vi "Get Joystick Values.vi"(8 "error in (no error)":errorcluster, 11 "Two Drivers in":refnum<class "Two Drivers.lvclass">) -> (0 "error out":errorcluster, 2 "Joystick Data":T1, 3 "Two Drivers out":refnum<class "Two Drivers.lvclass">)   [LabVIEW 2019, in "Joysticks.lvlib" / "Two Drivers.lvclass"]
doc: "Use this method to get the joystick values in a cluster you can use for your application.\n\nModify the Type Def that this VI resturns to fit the controls needed for the robot."
uses:
  Two Drivers.lvclass
  Joysticks.lvclass
  Controls/JoystickData.ctl
panel:
  in  "Sensitivity of Turret":dbl=45.0
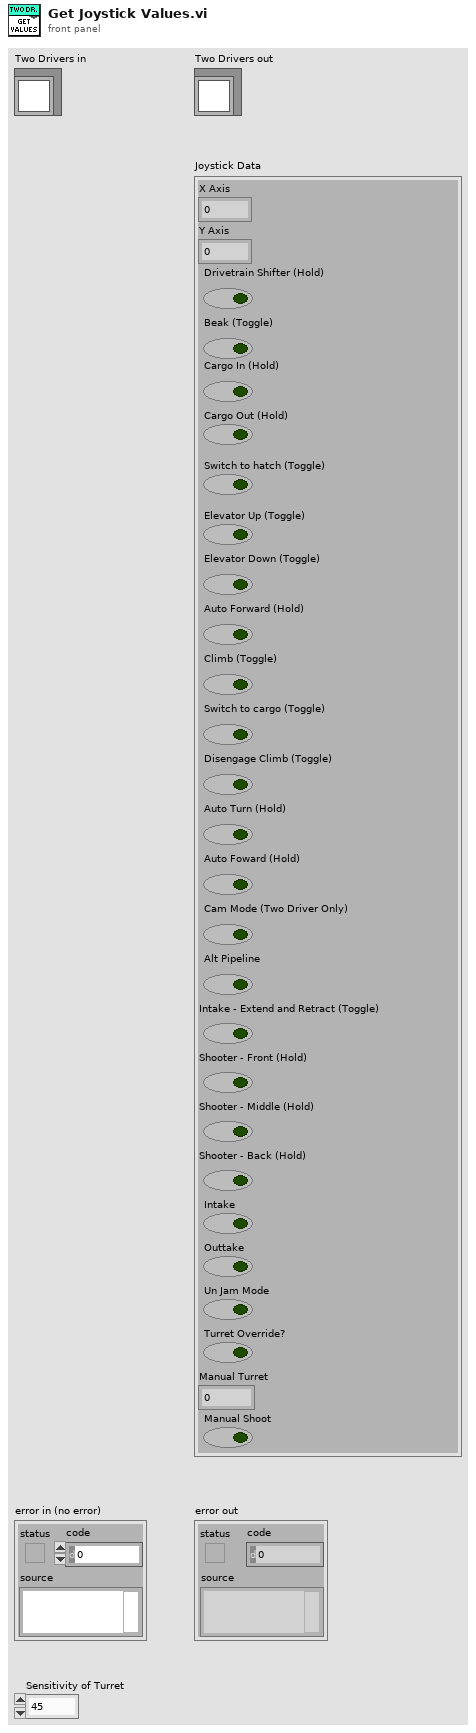
[diagram p1: front panel]
types:
  T1 = typedef "Joysticks.lvlib/Joysticks.lvclass/JoystickData.ctl" = cluster{"X Axis ":dbl, "Y Axis":dbl, "Drivetrain Shifter (Hold)":bool, "Beak (Toggle)":bool, "Cargo In (Hold)":bool, "Cargo Out (Hold)":bool, "Switch to hatch (Toggle)":bool, "Elevator Up (Toggle)":bool, "Elevator Down (Toggle)":bool, "Auto Forward (Hold)":bool, "Climb (Toggle)":bool, "Switch to cargo (Toggle)":bool, "Disengage Climb (Toggle)":bool, "Auto Turn (Hold)":bool, "Auto Foward (Hold)":bool, "Cam Mode (Two Driver Only)":bool, "Alt Pipeline":bool, "Intake - Extend and Retract (Toggle)":bool, "Shooter - Front (Hold)":bool, "Shooter - Middle (Hold)":bool, "Shooter - Back (Hold)":bool, "Intake":bool, "Outtake":bool, "Un Jam Mode":bool, "Turret Override?":bool, "Manual Turret":dbl, "Manual Shoot":bool}
  T2 = typedef "WPI_JoystickDevRef.ctl" = cluster{"Device":T3}
  T3 = typedef "WPI_JoystickDeviceEnum.ctl" = enum16{"USB 0", "USB 1", "USB 2", "USB 3", "USB 4", "USB 5"}
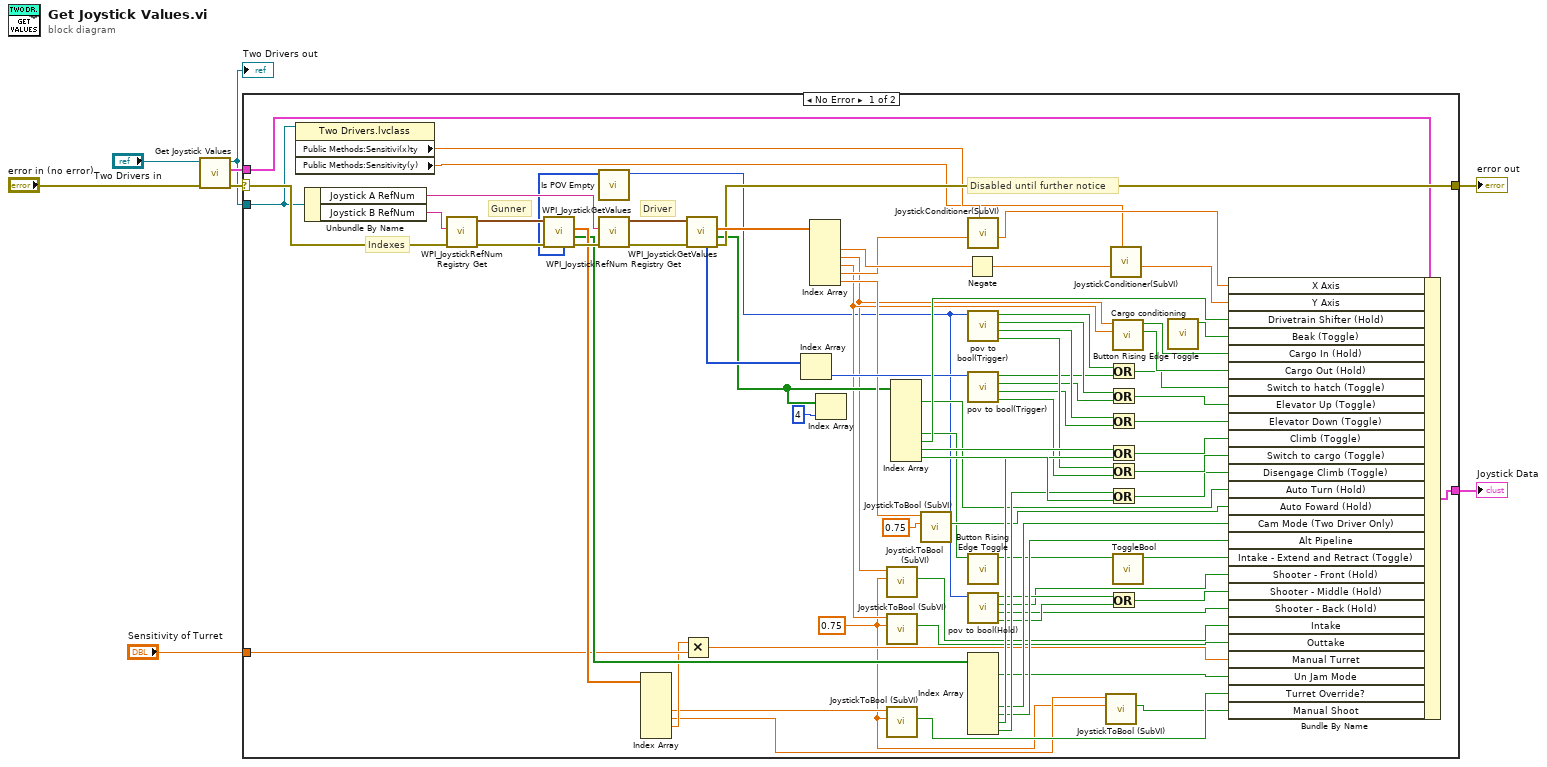
[diagram p0: block diagram]
diagram:
  n1 = call-parent "Get Joystick Values.vi"("error in (no error)"="error in (no error)", "Joysticks in"="Two Drivers in") -> ("error out"=w5:errorcluster, "Joystick Data"=w7:T1, "Joysticks out"=w3:refnum<class "Two Drivers.lvclass">)  [unwired: 7 in]
  "Two Drivers out" <- w3
  n2 = case shown="No Error" w5 {
    selector: w5 -> [w77 w86]
    tunnel: [w71 w86] -> w8
    tunnel: w3 -> [w56 _]
    tunnel: [w82 _] -> w2
    tunnel: w7 -> [w42 _]
    tunnel: "Sensitivity of Turret" -> [w14 _]
    frame No Error {
      w10 = 0.75 ("y")
      # "Indexes"
      # "Gunner"
      # "Driver"
      # "Disabled until further notice"
      n3 = property class="Two Drivers.lvclass"(reference=w56) -> ("Public Methods:Sensitivi(x)ty"=w55:dbl, "Public Methods:Sensitivity(y)"=w54:dbl)  [unwired: 1 in, 2 out]
      n4 = Unbundle By Name(w56) -> ("Joystick A RefNum"=w84:string, "Joystick B RefNum"=w74:string)
      n5 = call <vilib>:"WPI_JoystickRefNum Registry Get.vi"("error in (no error)"=w77, "refnum name"=w74) -> ("error out"=w76:errorcluster, "JoystickDevRef"=w78:T2)  [unwired: 8 in]
      n6 = call <vilib>:"WPI_JoystickGetValues.vi"("error in (no error)"=w76, "JoystickDevRef"=w78) -> ("error out"=w75:errorcluster, "Buttons"=w72:bool[], "Axes"=w73:dbl[], "POVs"=w30:i16[])  [unwired: 5 in, 1 out]
      n7 = call "Is POV Empty.vi"("POVs"=w30) -> ("Numeric"=w29:i16)  [unwired: 10 in]
      n8 = call <vilib>:"WPI_JoystickRefNum Registry Get.vi"("error in (no error)"=w75, "refnum name"=w84) -> ("error out"=w85:errorcluster, "JoystickDevRef"=w83:T2)  [unwired: 8 in]
      n9 = Index Array(array=w73) -> (element #3=w12:dbl, element #4=w11:dbl, element #5=w13:dbl)  [unwired: 6 in, 3 out]
      n10 = Multiply(x=w13, y=w14) -> (x*y=w15:dbl)
      n11 = call <vilib>:"WPI_JoystickGetValues.vi"("error in (no error)"=w85, "JoystickDevRef"=w83) -> ("error out"=w71:errorcluster, "Buttons"=w41:bool[], "Axes"=w81:dbl[], "POVs"=w70:i16[])  [unwired: 5 in, 1 out]
      n12 = Index Array(array=w70) -> (element=w67:i16)  [unwired: 1 in]
      n13 = Index Array(array=w81) -> (element #2=w79:dbl, element #3=w33:dbl, element #4=w34:dbl, element #5=w58:dbl, element #6=w48:dbl)  [unwired: 6 in, 1 out]
      n14 = Index Array(array=w41, index=4) -> ()  [unwired: 1 out]
      n15 = call "JoystickToBool (SubVI).vi"("Threshold"=w10, "Axis"=w33) -> ("Joy Forward"=w32:bool)  [unwired: 8 in, 1 out]
      n16 = call "JoystickToBool (SubVI).vi"("Threshold"=w10, "Axis"=w34) -> ("Joy Forward"=w31:bool)  [unwired: 8 in, 1 out]
      n17 = call "JoystickToBool (SubVI).vi"("Threshold"=w10, "Axis"=w12) -> ("Joy Forward"=w16:bool)  [unwired: 8 in, 1 out]
      n18 = Index Array(array=w41) -> (element #1=w43:bool, element #5=w35:bool, element #6=w80:bool, element #7=w68:bool, element #8=w53:bool)  [unwired: 8 in, 3 out]
      n19 = call "JoystickToBool (SubVI).vi"("Threshold"=0.75 ("y"), "Axis"=w48) -> ("Joy Forward"=w46:bool)  [unwired: 8 in, 1 out]
      n20 = Negate(x=w79) -> (-x=w60:dbl)
      n21 = call "JoystickConditioner(SubVI).vi"("Sensitivity"=w55, "joystick axis"=w58) -> ("output"=w57:dbl)  [unwired: 9 in]
      n22 = call "pov to bool(Trigger).vi"("Numeric"=w29) -> ("Left"=w25:bool, "Down"=w26:bool, "Up"=w27:bool, "Right"=w28:bool)  [unwired: 7 in]
      n23 = call "pov to bool(Trigger).vi"("Numeric"=w67) -> ("Left"=w21:bool, "Down"=w22:bool, "Up"=w23:bool, "Right"=w24:bool)  [unwired: 7 in]
      n24 = call "Button Rising Edge Toggle.vi"("Button"=w35) -> ("Rising edge?"=w18:bool)  [unwired: 10 in]
      n25 = call "pov to bool(Hold).vi"("Numeric"=w29) -> ("Left"=w38:bool, "Down"=w36:bool, "Up"=w37:bool, "Right"=w39:bool)  [unwired: 7 in]
      n26 = Index Array(array=w72) -> (element #1=w20:bool, element #5=w45:bool, element #6=w44:bool, element #7=w49:bool, element #8=w51:bool)  [unwired: 8 in, 3 out]
      n27 = call "JoystickToBool (SubVI).vi"("Threshold"=w10, "Axis"=w11) -> ("Joy Forward"=w9:bool)  [unwired: 8 in, 1 out]
      n28 = Or(x=w28, y=w24) -> (x .or. y?=w61:bool)
      n29 = Or(x=w27, y=w23) -> (x .or. y?=w62:bool)
      n30 = Or(x=w26, y=w22) -> (x .or. y?=w63:bool)
      n31 = Or(x=w68, y=w49) -> (x .or. y?=w50:bool)
      n32 = Or(x=w25, y=w21) -> (x .or. y?=w64:bool)
      n33 = Or(x=w51, y=w53) -> (x .or. y?=w52:bool)
      n34 = Or(x=w39, y=w38) -> (x .or. y?=w19:bool)
      n35 = call "JoystickConditioner(SubVI).vi"("Sensitivity"=w54, "joystick axis"=w60) -> ("output"=w59:dbl)  [unwired: 9 in]
      n36 = call "Cargo conditioning.vi"("Cargo Out (Axis)"=w34, "Cargo In (Axis)"=w33) -> ("Cargo Out (Hold)"=w65:bool, "Cargo In (Hold)"=w66:bool)  [unwired: 8 in]
      n37 = call "ToggleBool.vi"("Boolean"=w18) -> ("toggled bool"=w17:bool)  [unwired: 10 in]
      n38 = call "Button Rising Edge Toggle.vi"() -> ("Rising edge?"=w69:bool)  [unwired: 11 in]
      n39 = Bundle By Name(cluster=w42, "X Axis"=w57, "Y Axis"=w59, "Drivetrain Shifter (Hold)"=w80, "Beak (Toggle)"=w69, "Cargo In (Hold)"=w66, "Cargo Out (Hold)"=w65, "Switch to hatch (Toggle)"=w61, "Elevator Up (Toggle)"=w62, "Elevator Down (Toggle)"=w63, "Climb (Toggle)"=w50, "Switch to cargo (Toggle)"=w64, "Disengage Climb (Toggle)"=w52, "Auto Turn (Hold)"=w43, "Auto Foward (Hold)"=w46, "Cam Mode (Two Driver Only)"=w45, "Alt Pipeline"=w44, "Intake - Extend and Retract (Toggle)"=w17, "Shooter - Front (Hold)"=w37, "Shooter - Middle (Hold)"=w19, "Shooter - Back (Hold)"=w36, "Intake"=w32, "Outtake"=w31, "Manual Turret"=w15, "Un Jam Mode"=w20, "Turret Override?"=w16, "Manual Shoot"=w9) -> (w82:T1)
    }
    frame Error {
    }
  }
  "error out" <- w8
  "Joystick Data" <- w2
